vi "ex_CreateSignalChunkString.vi"(0 "Signals":waveform(dbl)[](array[waveform]), 1 "nPoints array":i32[](array[numeric]), 2 "max nPoints index":i32, 3 "Decimal Separator":string="%;%g", 5 "X0 array":timestamp[](array[timestamp])=[timestamp(0 s since 1904-01-01), timestamp(0 s since 1904-01-01)] format="%<%X\n%x>T", 7 "first?":bool, 9 "dX array":dbl[](array[numeric]) format="%.2f", 11 "x_columns":u16(ring)=2 items=["None", "One", "Multiple"], 12 "delimiter (Tab)":string="\t", 13 "comment":string, 14 "time format":string) -> (4 "spreadsheet string":string)   [LabVIEW 2020]
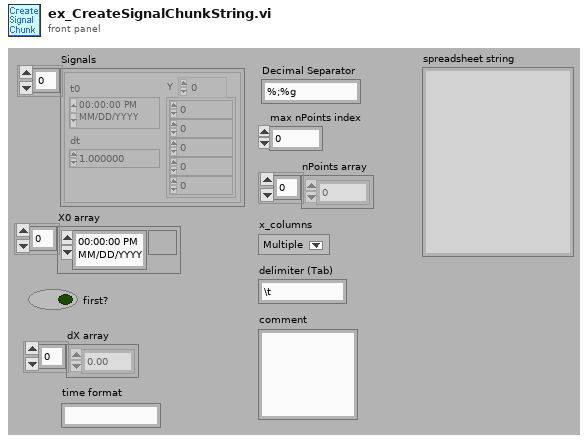
[diagram p1: front panel]
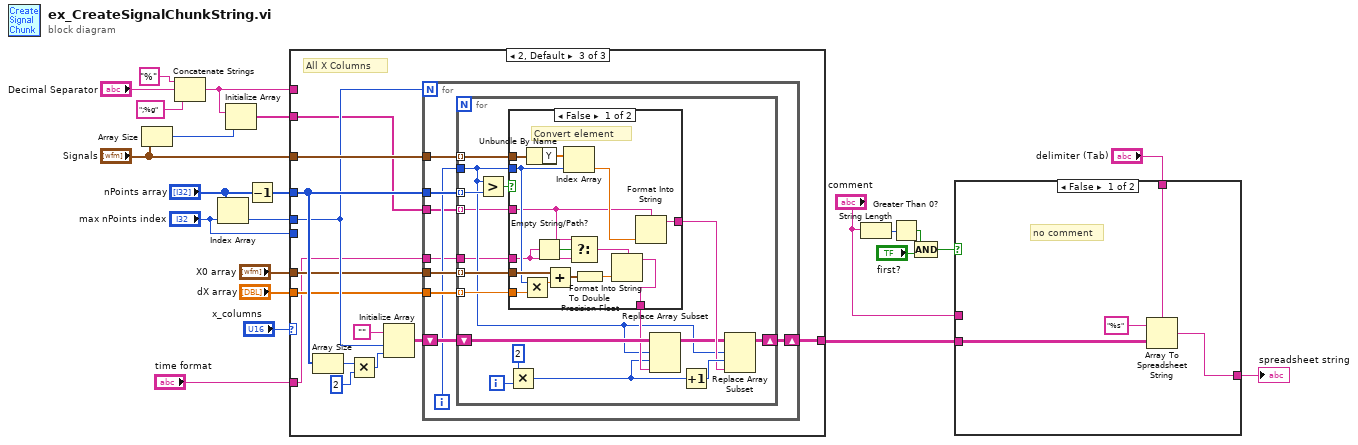
[diagram p0: block diagram]
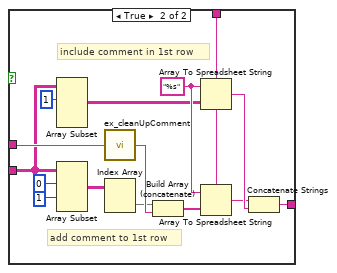
[diagram p2: hidden frame]
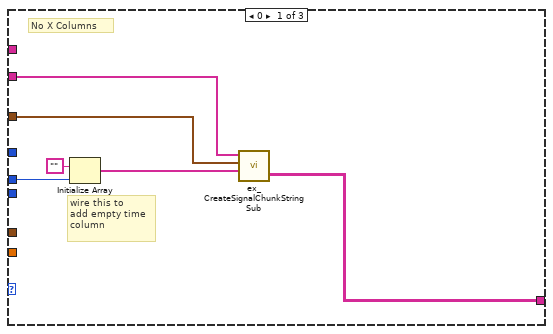
[diagram p3: hidden frame]
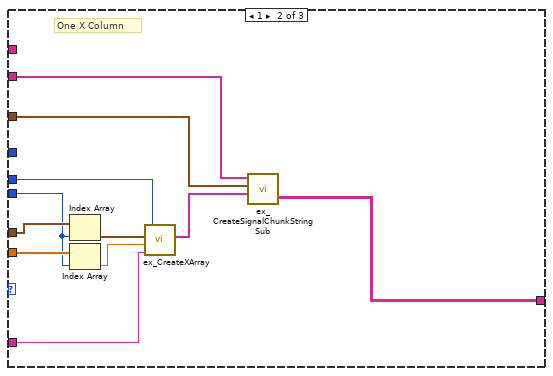
[diagram p4: hidden frame]
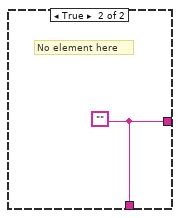
[diagram p5: hidden frame]
diagram:
  n1 = Array Size(array="Signals") -> (size(s)=w16:i32)
  n2 = Concatenate Strings("%" ("string"), "Decimal Separator", ";%g" ("string")) -> (w1:string)
  n3 = Index Array(array="nPoints array", index="max nPoints index") -> (element=w22:i32)
  n4 = Initialize Array(w1, w16) -> (w17:string[])
  n5 = Decrement(x="nPoints array") -> (x-1=w21:i32[])
  n6 = case shown="2, Default" "x_columns" {
    tunnel: "Signals" -> [w29 w31 w53]
    tunnel: w22 -> [w25 w40 w47]
    tunnel: w21 -> [_ _ w52]
    tunnel: [w28 w32 w46] -> w8
    tunnel: "X0 array" -> [_ w37 w44]
    tunnel: "dX array" -> [_ w36 w45]
    tunnel: "max nPoints index" -> [_ w35 _]
    tunnel: w17 -> [w27 w33 w43]
    tunnel: "time format" -> [_ w30 w41]
    tunnel: w1 -> [_ _ _]
    frame 0 {
      # "wire this to\nadd empty time\ncolumn"
      # "No X Columns"
      n7 = Initialize Array("", w25) -> (w24:string[])
      n8 = call <vilib>:"ex_CreateSignalChunkStringSub.vi"("data"=w24, "Signals"=w29, "format"=w27) -> ("Array"=w28:string[][])  [unwired: 4 out]
    }
    frame 1 {
      # "One X Column"
      n9 = Index Array(array=w37, index=w35) -> (element=w38:timestamp)
      n10 = Index Array(array=w36, index=w35) -> (element=w39:dbl)
      n11 = call <vilib>:"ex_CreateXArray.vi"("time format"=w30, "delta x"=w39, "x0"=w38, "samples"=w40) -> ("x array"=w34:string[])  [unwired: 3 out]
      n12 = call <vilib>:"ex_CreateSignalChunkStringSub.vi"("data"=w34, "Signals"=w31, "format"=w33) -> ("Array"=w32:string[][])  [unwired: 4 out]
    }
    frame 2, Default {
      # "All X Columns"
      n13 = Array Size(array=w52) -> (size(s)=w50:i32)
      n14 = Multiply(x=w50, y=2) -> (x*y=w42:i32)
      n15 = Initialize Array("", w47, w42) -> (w48:string[][])
      n16 = for {
        N: w47 -> [_]
        tunnel: w53 -> [w61]
        tunnel: w52 -> [w62]
        shift-right: [w60] -> w46
        shift-left: w48 -> [w58]
        tunnel: w45 -> [w59]
        tunnel: w44 -> [w57]
        tunnel: w43 -> [w55]
        tunnel: w41 -> [w54]
        i -> [w56]
        n17 = for {
          tunnel: w62 -> [w79] mode=indexing
          tunnel: w61 -> [w77] mode=indexing
          shift-right: [w64] -> w60
          shift-left: w58 -> [w76]
          tunnel: w56 -> [w67]
          tunnel: w57 -> [w74] mode=indexing
          tunnel: w59 -> [w73] mode=indexing
          tunnel: w55 -> [w65] mode=indexing
          tunnel: w54 -> [w63]
          i -> [w66]
          n18 = Greater?(x=w67, y=w79) -> (0:w78:bool)
          n19 = Multiply(x=2, y=w66) -> (x*y=w68:i32)
          n20 = case shown="False" w78 {
            tunnel: w77 -> [w94 _]
            tunnel: w67 -> [w90 _]
            tunnel: [w87 w95] -> w72
            tunnel: w74 -> [w92 _]
            tunnel: w73 -> [w91 _]
            tunnel: [w86 w95] -> w71
            tunnel: w65 -> [w85 _]
            tunnel: w63 -> [w83 _]
            frame False {
              # "Convert element"
              n21 = Multiply(x=w90, y=w91) -> (x*y=w89:dbl)
              n22 = Unbundle By Name(w94) -> ("Y"=w93:dbl[])
              n23 = Empty String/Path?(string/path=w83) -> (empty?=w84:bool)
              n24 = Add(x=w92, y=w89) -> (x+y=w81:timestamp)
              n25 = Index Array(array=w93, index=w90) -> (element=w88:dbl)
              n26 = Select(t=w85, s=w84, f=w83) -> (s? t:f=w82:string)
              n27 = To Double Precision Float(number=w81) -> (double precision float=w80:dbl)
              n28 = Format Into String(format string=w82, w80) -> (resulting string=w86:string)  [unwired: 2 in, 1 out]
              n29 = Format Into String(format string=w85, w88) -> (resulting string=w87:string)  [unwired: 2 in, 1 out]
            }
            frame True {
              w95 = ""
              # "No element here"
            }
          }
          n30 = Replace Array Subset(array=w76, new element=w71, index (row)=w67, index (col)=w68) -> (w70:string[][])
          n31 = Increment(x=w68) -> (x+1=w75:i32)
          n32 = Replace Array Subset(array=w70, new element=w72, index (row)=w67, index (col)=w75) -> (w64:string[][])
        }
      }
    }
  }
  n33 = String Length(string="comment") -> (length=w14:i32)
  n34 = Greater Than 0?(x=w14) -> (x > 0?=w12:bool)
  n35 = Compound Arithmetic op=AND(w12, "first?") -> (w13:bool)
  n36 = case shown="False" w13 {
    tunnel: [w97 w112] -> w9
    tunnel: "delimiter (Tab)" -> [w98 w100]
    tunnel: "comment" -> [_ w104]
    tunnel: w8 -> [w96 w101]
    frame False {
      # "no comment"
      n37 = Array To Spreadsheet String(delimiter (Tab)=w98, array=w96, 3:"%s" ("format (%.3f)")) -> (spreadsheet string=w97:string)
    }
    frame True {
      w113 = "%s" ("format (%.3f)")
      # "include comment in 1st row"
      # "add comment to 1st row"
      n38 = Array Subset(array=w101, index (row)=1 ("index")) -> (w103:string[][])  [unwired: 3 in]
      n39 = Array Subset(array=w101, index (row)=0 ("index"), length (row)=1 ("length")) -> (w106:string[][])  [unwired: 2 in]
      n40 = call <vilib>:"ex_cleanUpComment.vi"("comment"=w104) -> ("output"=w105:string)
      n41 = Index Array(array=w106) -> (element=w102:string[])  [unwired: 2 in]
      n42 = Build Array (concatenate)(w102, w105) -> (w107:string[])
      n43 = Array To Spreadsheet String(delimiter (Tab)=w100, array=w103, 3:w113) -> (spreadsheet string=w114:string)
      n44 = Array To Spreadsheet String(delimiter (Tab)=w100, array=w107, 3:w113) -> (spreadsheet string=w111:string)
      n45 = Concatenate Strings(w111, w114) -> (w112:string)
    }
  }
  "spreadsheet string" <- w9
